vi "JSONRPC-Info.vi"(8 "error in (no error)":errorcluster, 11 "expId":string) -> (0 "error out":errorcluster, 3 "result":string)   [LabVIEW 2019]
doc: "Invokes the actual implementation of a RIP <b>method</b>."
uses:
  Configuration/Global_Configurations.vi
panel:
  # "Info"
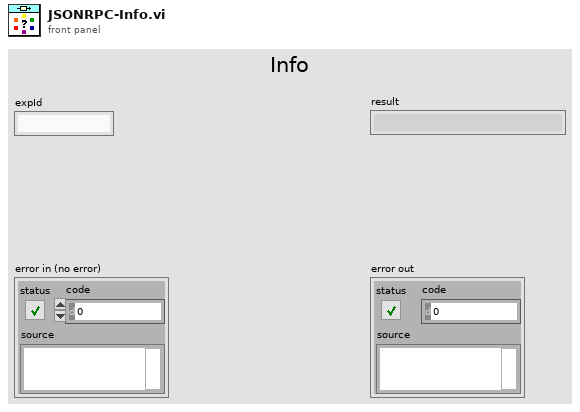
[diagram p1: front panel]
types:
  T1 = cluster{"Path":path, "Name":string, "Authors":string, "Keywords":string, "Description":string, "Cameras":cluster{"Base URL":string, "Path":string, "Name":string}[], "Sampling":cluster{"Sampled Variable":string, "Delta":dbl}[], "Sampling Freq":u32}[]
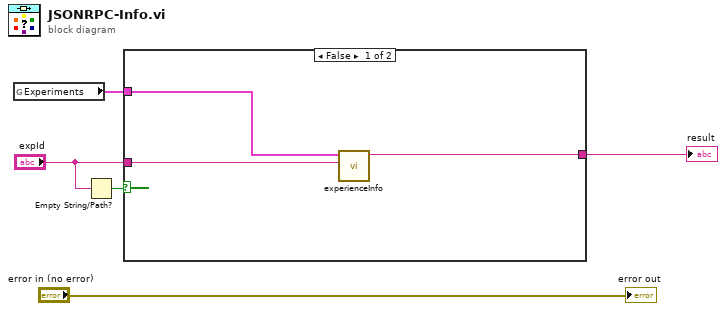
[diagram p0: block diagram]
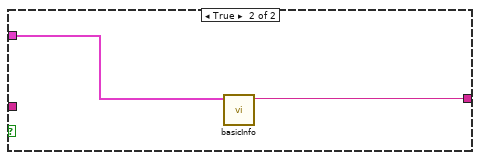
[diagram p2: hidden frame]
diagram:
  n1 = global read "Global_Configurations.vi" "Experiments"() -> (w2:T1)
  n2 = Empty String/Path?(string/path="expId") -> (empty?=w4:bool)
  n3 = case shown="False" w4 {
    tunnel: "expId" -> [w8 _]
    tunnel: [w7 w10] -> w1
    tunnel: w2 -> [w6 w9]
    frame False {
      n4 = call "experienceInfo.vi"("info in"=w8, "Experiments"=w6) -> ("info out"=w7:string)  [unwired: 9 in]
    }
    frame True {
      n5 = call "basicInfo.vi"("Experiments"=w9) -> ("String"=w10:string)  [unwired: 10 in]
    }
  }
  "result" <- w1
  "error out" <- "error in (no error)"
